vi "FPGA.vi"() -> ()   [LabVIEW 2013]
uses:
  PMUmeasurements.ctl
  FreqEstimator.ctl
  ToFPGA.ctl
  <vilib>/rvi/FXPMathLib/FxpSinAndCos/subVIs/nifxpmath_SinAndCos_SimConfig.ctl
  <vilib>/rvi/Emulation/niFpgaSctlEmulationGetInTimedLoop.vi
  <vilib>/rvi/Emulation/niFpgaEmulationReportErrorSimple.vi
  <vilib>/rvi/Emulation/niFpgaGetClockAttributes.vi
  <vilib>/rvi/eio/common/nirviEmuTemplateMethod_errors.vi
  <vilib>/rvi/FXPMathLib/FxpSinAndCos/simVIs/DllFxpSinAndCosTemp_sub.vi
  <vilib>/rvi/Emulation/niFpgaCriticalErrorInLSC.vi
  <vilib>/eio/EIONode/EIONode.xnode
  <vilib>/rvi/FXPMathLib/FxpSinAndCos/XNode/nifxpmath_SinAndCos.xnode
panel:
  in  "Scaling":sgl
  out "Loop period monitoring":u8
  out "The output signals":T1
  out "FPGA Error Out":errorcluster
  in  "Alpha":sgl
  in  "Frequency Estimator Settings":T2={"Parameters"={"Ts"=5e-05, "kappaav"=0.625, "kappaph"=0.5762, "mu"=0.7086}}
  in  "Freq of Osc":sgl=0.64
  in  "PMU measurments":T3
  in  "stop":bool
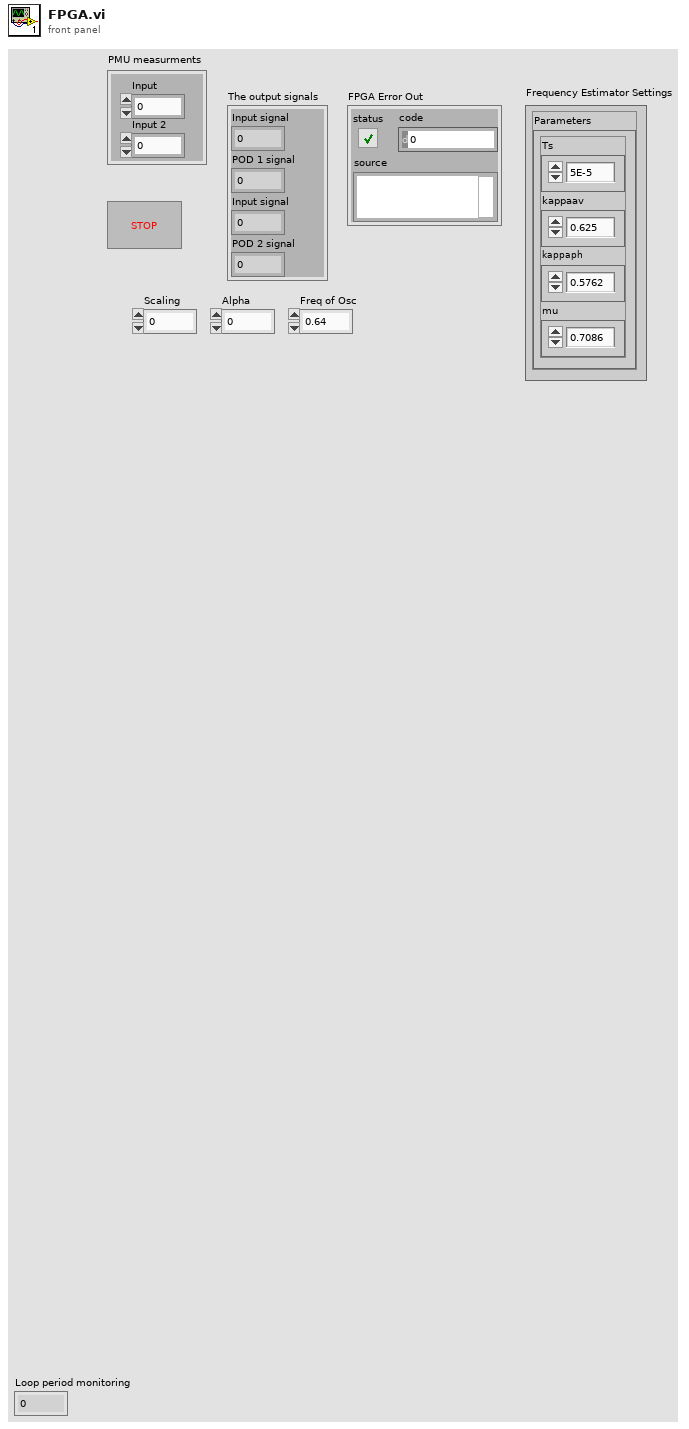
[diagram p1: front panel]
types:
  T1 = typedef "ToFPGA.ctl" = cluster{"Input signal":sgl, "POD 1 signal":sgl, "Input signal":sgl, "POD 2 signal":sgl}
  T2 = typedef "FreqEstimator.ctl" = cluster{"Parameters":cluster{"Ts":sgl, "kappaav":sgl, "kappaph":sgl, "mu":sgl}}
  T3 = typedef "PMUmeasurements.ctl" = cluster{"Input":sgl, "Input 2":sgl}
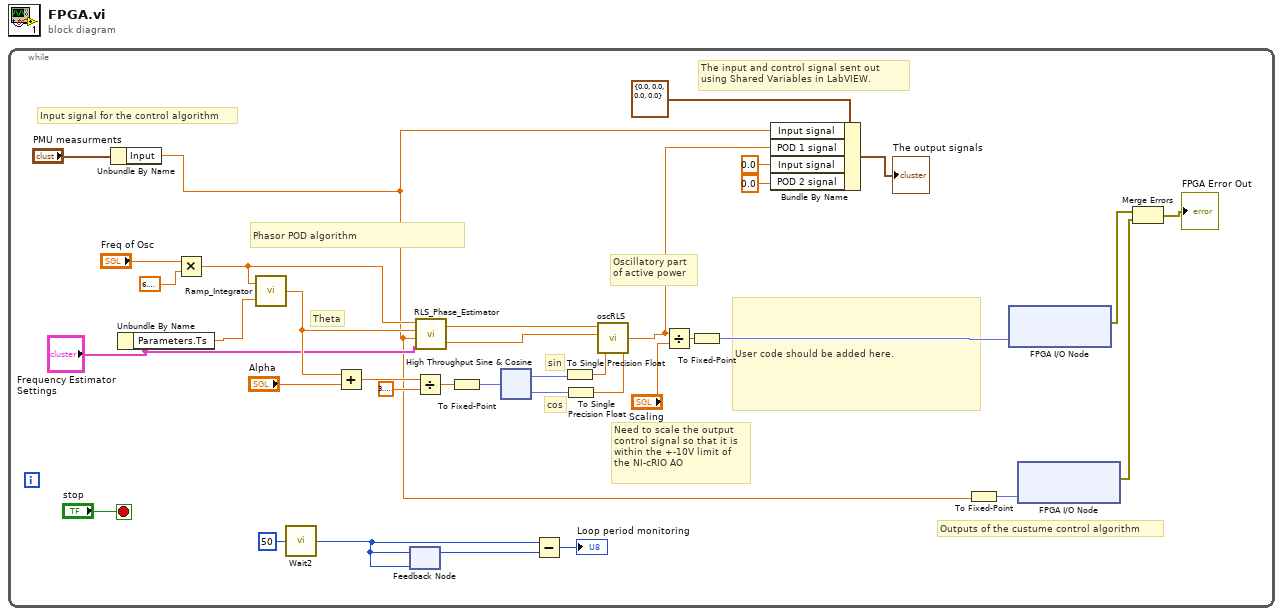
[diagram p0: block diagram]
diagram:
  n1 = while {
    stop <- "stop" stop-if-true
    # "Phasor POD algorithm"
    # "Need to scale the output \ncontrol signal so that it is \nwithin the +-10V limit of \nthe NI-cRIO AO"
    # "Outputs of the custume control algorithm"
    # "User code should be added here."
    # "The input and control signal sent out using Shared Variables in LabVIEW."
    # "Input signal for the control algorithm"
    # "Oscillatory part \nof active power"
    # "Theta"
    # "cos"
    # "sin"
    n2 = Unbundle By Name("PMU measurments") -> ("Input"=w4:sgl)
    n3 = Unbundle By Name("Frequency Estimator Settings") -> ("Parameters.Ts"=w9:sgl)
    n4 = Multiply(x="Freq of Osc", y=sgl 6.2831855) -> (x*y=w31:sgl)
    n5 = call "Ramp_Integrator.vi"("tsample"=w9, "w"=w31) -> ("theta"=w19:sgl)
    n6 = call "Wait2"("Count(uSec)"=u8 50) -> ("Tick Count(uSec)"=w10:u8)
    n7 = Add(x=w19, y="Alpha") -> (x+y=w18:sgl)
    n8 = feedback #1(w10) -> (w11:u8)
    n9 = feedback-in #1(w10) -> ()
    n10 = Divide(x=w18, y=sgl 3.1415927) -> (x/y=w29:sgl)
    n11 = call "RLS_Phase_Estimator.vi"("Frequency Estimator Settings"="Frequency Estimator Settings", "u"=w4, "theta"=w19, "wcs"=w31) -> ("uphq"=w22:sgl, "uphd"=w23:sgl)
    n12 = To Fixed-Point(number=w29) -> (fixed-point=w28:fxp<+/-,20,5>)  [unwired: 1 in]
    n13 = xnode "High Throughput Sine & Cosine"("x (pi)"=w28) -> ("sin(x)"=w27:fxp<+/-,16,2>, "cos(x)"=w26:fxp<+/-,16,2>)
    n14 = Subtract(x=w10, y=w11) -> (x-y=→"Loop period monitoring":u8)
    n15 = To Single Precision Float(number=w27) -> (single precision float=w25:sgl)
    n16 = To Single Precision Float(number=w26) -> (single precision float=w24:sgl)
    n17 = call "oscRLS.vi"("u4"=w25, "u3"=w24, "u2"=w22, "u1"=w23) -> ("f(u)"=w2:sgl)
    n18 = Divide(x=w2, y="Scaling") -> (x/y=w7:sgl)
    n19 = To Fixed-Point(number=w7) -> (fixed-point=w13:fxp<+/-,20,5>)  [unwired: 1 in]
    n20 = Bundle By Name(cluster=T1 {"Input signal"=0.0, "POD 1 signal"=0.0, "Input signal"=0.0, "POD 2 signal"=0.0}, "Input signal"=w4, "POD 1 signal"=w2, "Input signal"=sgl 0.0 ("Empty"), "POD 2 signal"=sgl 0.0 ("Empty")) -> (→"The output signals":T1)
    n21 = To Fixed-Point(number=w4) -> (fixed-point=w21:fxp<+/-,20,5>)  [unwired: 1 in]
    n22 = xnode "FPGA I/O Node"("Mod1/AO1"=w13) -> ("error out"=w17:errorcluster)  [unwired: 2 in, 1 out]
    n23 = xnode "FPGA I/O Node"("Mod1/AO0"=w21) -> ("error out"=w16:errorcluster)  [unwired: 2 in, 1 out]
    n24 = Merge Errors(w17, w16) -> (→"FPGA Error Out":errorcluster)
  }
